vi "FlipFlop.vi"() -> ()   [LabVIEW 2012]
panel:
  out "Q Roof":bool
  out "Q":bool
  in  "S":bool
  in  "R":bool
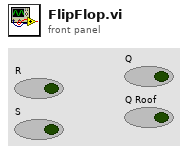
[diagram p1: front panel]
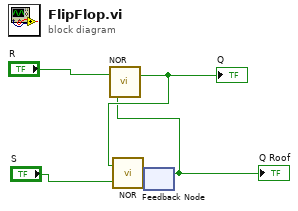
[diagram p0: block diagram]
diagram:
  n1 = feedback #1() -> (w1:bool)  [unwired: 1 in]
  "Q Roof" <- w1
  n2 = call "NOR.vi"("b"=w1, "a"="R") -> ("x"=w3:bool)
  "Q" <- w3
  n3 = call "NOR.vi"("b"="S", "a"=w3) -> ("x"=w2:bool)
  n4 = feedback-in #1(w2) -> ()
